vi "Read Module Reporting.vi"(7 "Module ID":string, 8 "error in":errorcluster, 11 "Standard Engine Repo Data in":refnum<class "Standard Engine Configuration.lvclass">) -> (0 "error out":errorcluster, 2 "error tag":string, 3 "Standard Engine Repo Data out":refnum<class "Standard Engine Configuration.lvclass">)   [LabVIEW 2013, in "Standard Engine Configuration.lvclass"]
doc: "Returns error reporting information for a specific module configured using the 'enable error reporting.vi'."
uses:
  Standard Engine Configuration.lvclass
  Standard Engine Configuration.lvclass/Standard Engine Configuration.ctl
  <vilib>/NI/Configuration Framework/NISE_CEF_TreeControl.lvlib
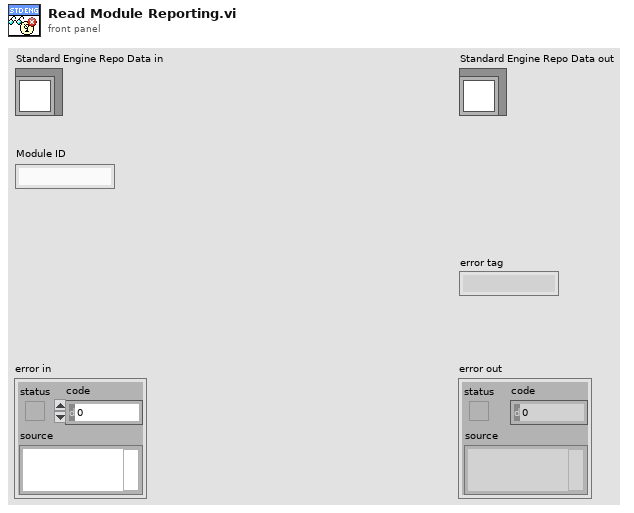
[diagram p1: front panel]
types:
  T1 = typedef "Standard Engine Configuration.lvclass/Module Specific Configuration.ctl" = cluster{"Module ID":string, "Module Decimation":T2, "error tag":string, "error responses":T3}
  T2 = typedef "Standard Engine Configuration.lvclass/Module Decimation.ctl" = cluster{"Decimation":u16, "Offset":u16, "sort order":i32, "async?":bool}
  T3 = typedef "Standard Engine Configuration.lvclass/error responses.ctl" = cluster{"unknown":T4, "trivial":T4, "critical":T4, "recoverable":T4}
  T4 = typedef "Standard Engine Configuration.lvclass/error options.ctl" = cluster{"clear":bool, "notify":bool, "remove module":bool, "abort engine":bool, "go to safe state":bool, "recover module":bool}
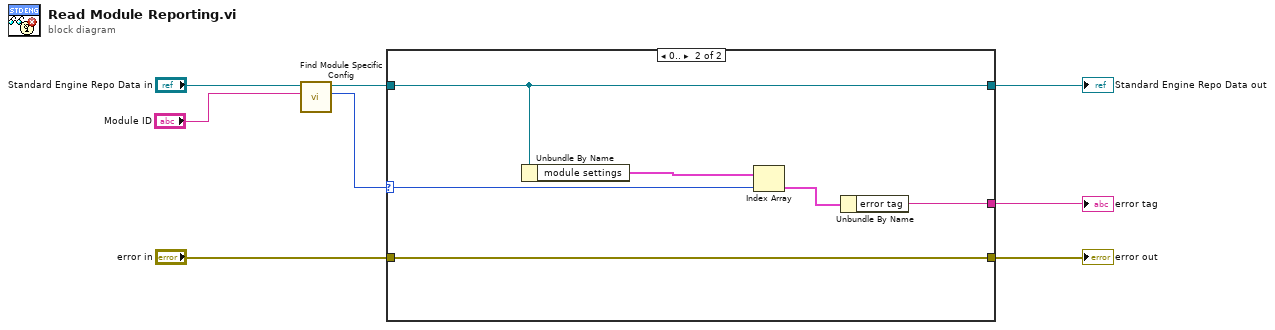
[diagram p0: block diagram]
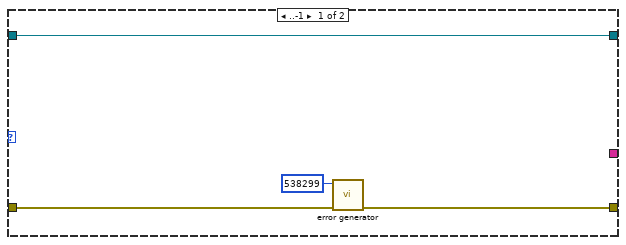
[diagram p2: hidden frame]
diagram:
  n1 = call "Find Module Specific Config.vi"("Module ID"="Module ID", "Standard Engine Repo Data in"="Standard Engine Repo Data in") -> ("Index"=w1:i32, "Standard Engine Repo Data out"=w2:refnum<class "Standard Engine Configuration.lvclass">)  [unwired: 8 in]
  n2 = case shown="0.." w1 {
    selector: w1 -> [_ w15]
    tunnel: w2 -> [w12 w16]
    tunnel: "error in" -> [w11 w14]
    tunnel: [w10 w14] -> w6
    tunnel: [w12 w16] -> w4
    tunnel: [_ w13] -> w3
    frame ..-1 {
      n3 = call <vilib>:"error generator.vi"("error in"=w11, "error code (0)"=538299) -> ("error out"=w10:errorcluster)  [unwired: 7 in]
    }
    frame 0.. {
      n4 = Unbundle By Name(w16) -> ("module settings"=w18:T1[])
      n5 = Index Array(array=w18, index=w15) -> (element=w17:T1)
      n6 = Unbundle By Name(w17) -> ("error tag"=w13:string)
    }
  }
  "error out" <- w6
  "Standard Engine Repo Data out" <- w4
  "error tag" <- w3
